vi "sub vi - QPD channels.vi"() -> (2 "QPD Channels":tag="Dev1/ai21,Dev1/ai22,Dev1/ai23")   [LabVIEW 2010]
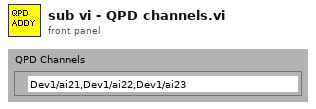
[diagram p1: front panel]
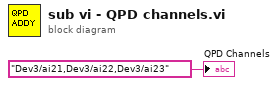
[diagram p0: block diagram]
diagram:
  "QPD Channels" <- tag "Dev3/ai21,Dev3/ai22,Dev3/ai23" ("physical channels")
